vi "programa1.vi"() -> ()   [LabVIEW 2011]
panel:
  out "Multiplicar":dbl
  out "División":dbl
  out "Resta":dbl
  out "Suma":dbl
  in  "Numero 2":dbl
  in  "Numero 1":dbl
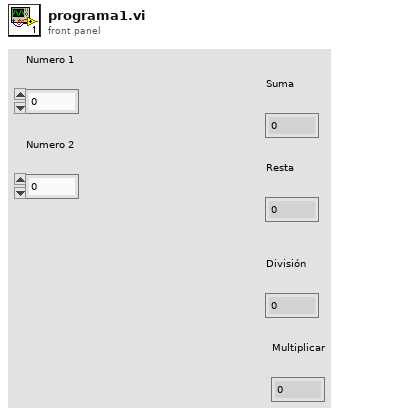
[diagram p1: front panel]
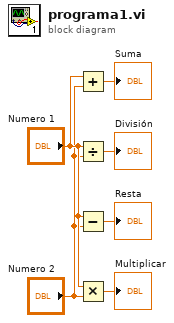
[diagram p0: block diagram]
diagram:
  n1 = Add(x="Numero 1", y="Numero 2") -> (x+y=→"Suma":dbl)
  n2 = Divide(x="Numero 1", y="Numero 2") -> (x/y=→"División":dbl)
  n3 = Subtract(x="Numero 1", y="Numero 2") -> (x-y=→"Resta":dbl)
  n4 = Multiply(x="Numero 1", y="Numero 2") -> (x*y=→"Multiplicar":dbl)
